vi "Convert GPS to Meters.vi"() -> ()   [LabVIEW 2009]
uses:
  TypeDefs/Sensor TypeDefs/GPS Data.ctl
panel:
  out "Distance":dbl
  in  "End GPS point":T1 {"Longitude" format="%#_14g"; "Latitude" format="%#_14g"}
  in  "Start GPS point":T1 {"Longitude" format="%#_14g"; "Latitude" format="%#_14g"}
  # "Uses haversine formula to convert GPS to meters"
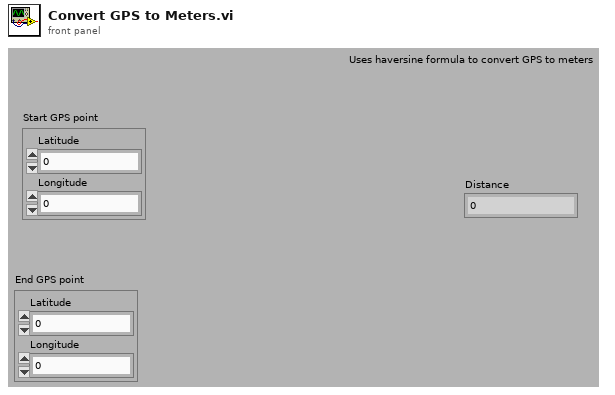
[diagram p1: front panel]
types:
  T1 = typedef "GPS Data.ctl" = cluster{"Latitude":dbl, "Longitude":dbl}
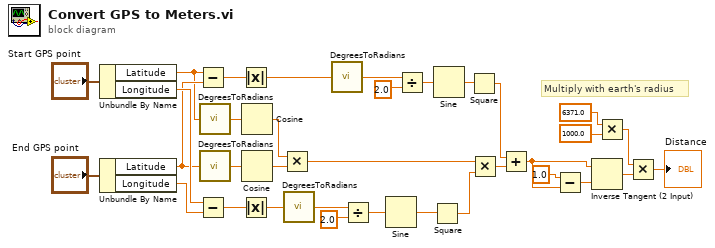
[diagram p0: block diagram]
diagram:
  # "Multiply with earth's radius"
  n1 = Unbundle By Name("Start GPS point") -> ("Latitude"=w10:dbl, "Longitude"=w30:dbl)
  n2 = Unbundle By Name("End GPS point") -> ("Latitude"=w12:dbl, "Longitude"=w29:dbl)
  n3 = Subtract(x=w10, y=w12) -> (x-y=w31:dbl)
  n4 = Subtract(x=w30, y=w29) -> (x-y=w28:dbl)
  n5 = call "DegreesToRadians.vi"("Degrees"=w10) -> ("Radians"=w9:dbl)
  n6 = call "DegreesToRadians.vi"("Degrees"=w12) -> ("Radians"=w11:dbl)
  n7 = Absolute Value(x=w31) -> (abs(x)=w27:dbl)
  n8 = Absolute Value(x=w28) -> (abs(x)=w26:dbl)
  n9 = Cosine(x=w9) -> (cos(x)=w16:dbl)
  n10 = Cosine(x=w11) -> (cos(x)=w15:dbl)
  n11 = Multiply(x=w16, y=w15) -> (x*y=w14:dbl)
  n12 = call "DegreesToRadians.vi"("Degrees"=w26) -> ("Radians"=w18:dbl)
  n13 = call "DegreesToRadians.vi"("Degrees"=w27) -> ("Radians"=w24:dbl)
  n14 = Divide(x=w18, y=2.0) -> (x/y=w19:dbl)
  n15 = Sine(x=w19) -> (sin(x)=w21:dbl)
  n16 = Divide(x=w24, y=2.0) -> (x/y=w22:dbl)
  n17 = Square(x=w21) -> (x^2=w13:dbl)
  n18 = Sine(x=w22) -> (sin(x)=w25:dbl)
  n19 = Square(x=w25) -> (x^2=w17:dbl)
  n20 = Multiply(x=w14, y=w13) -> (x*y=w8:dbl)
  n21 = Add(x=w17, y=w8) -> (x+y=w6:dbl)
  n22 = Subtract(x=1.0 ("y"), y=w6) -> (x-y=w5:dbl)
  n23 = Inverse Tangent (2 Input)(1:w5, 2:w6) -> (0:w3:dbl)
  n24 = Multiply(x=6371.0, y=1000.0) -> (x*y=w4:dbl)
  n25 = Multiply(x=w4, y=w3) -> (x*y=→"Distance":dbl)
